vi "Message Name.vi"(8 "error in (no error)":errorcluster, 9 "Text":string, 10 "Message Stack in":refnum<queue>, 11 "ProtoParser in":refnum<class "ProtoParser.lvclass">) -> (0 "error out":errorcluster, 2 "Message Name":string, 3 "ProtoParser out":refnum<class "ProtoParser.lvclass">)   [LabVIEW 2020, in "LV-Protoc.lvlib" / "ProtoParser.lvclass"]
uses:
  ProtoParser.lvclass
  LV-Proto/Message.ctl
  LV-Proto/Field.ctl
  LV-Proto/Type.ctl
  LV-Proto/Proto Type.ctl
  LV-Proto/LV-Proto.lvlib
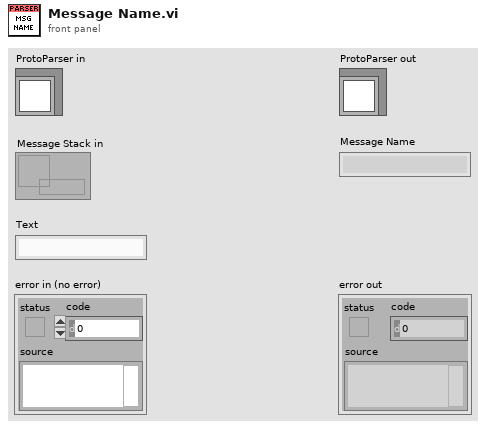
[diagram p1: front panel]
types:
  T1 = typedef "LV-Proto.lvlib/Message.ctl" = cluster{"Name":string, "Fields":T2[], "Reserved Numbers":u32[], "Reserved Names":string[]}
  T2 = typedef "LV-Proto.lvlib/Field.ctl" = cluster{"Name":string, "Number":u32, "Optional":bool, "Repeated":bool, "Type":T3, "Key Type":T3, "Value Type":T3}
  T3 = typedef "LV-Proto.lvlib/Type.ctl" = cluster{"Type":T4, "Subtype":string}
  T4 = typedef "LV-Proto.lvlib/Proto Type.ctl" = enum16{"UNKNOWN", "double", "float", "int32", "int64", "uint32", "uint64", "sint32", "sint64", "fixed32", "fixed64", "sfixed32", "sfixed64", "bool", "string", "bytes", "enum", "map", "message"}
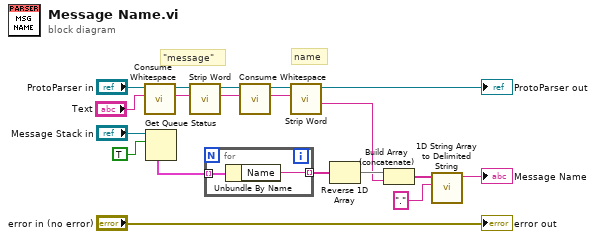
[diagram p0: block diagram]
diagram:
  # "name"
  # "\"message\""
  n1 = call "Consume Whitespace.vi"("String"="Text", "ProtoParser in"="ProtoParser in") -> ("Remaining"=w7:string, "ProtoParser out"=w10:refnum<class "ProtoParser.lvclass">)  [unwired: 7 in, 1 out]
  n2 = Get Queue Status(queue="Message Stack in", return elements? (F)=TRUE) -> (elements=w17:T1[])  [unwired: 1 in, 7 out]
  n3 = call "Strip Word.vi"("String"=w7, "ProtoParser in"=w10) -> ("Remaining"=w5:string, "ProtoParser out"=w8:refnum<class "ProtoParser.lvclass">)  [unwired: 6 in, 2 out]
  n4 = for {
    tunnel: w17 -> [w21] mode=indexing
    tunnel: [w20] -> w16 mode=indexing
    n5 = Unbundle By Name(w21) -> ("Name"=w20:string)
  }
  n6 = call "Consume Whitespace.vi"("String"=w5, "ProtoParser in"=w8) -> ("Remaining"=w3:string, "ProtoParser out"=w6:refnum<class "ProtoParser.lvclass">)  [unwired: 7 in, 1 out]
  n7 = call "Strip Word.vi"("String"=w3, "ProtoParser in"=w6) -> ("Word"=w2:string, "ProtoParser out"=→"ProtoParser out":refnum<class "ProtoParser.lvclass">)  [unwired: 6 in, 2 out]
  n8 = Reverse 1D Array(array=w16) -> (reversed array=w15:string[])
  n9 = Build Array (concatenate)(w15, w2) -> (w1:string[])
  n10 = call <vilib>:"1D String Array to Delimited String.vi"("delimiter"=".", "string array"=w1) -> ("delimited string"=→"Message Name":string)  [unwired: 9 in]
  "error out" <- "error in (no error)"
